vi "Dashboard Loop.vi"(10 "connection ID":refnum<k16>) -> ()   [LabVIEW 2016]
uses:
  Common Code/Intake Mode.ctl
  Common Code/Intake Commands.ctl
  Common Code/Intake Status Cluster.ctl
  Common Code/Climb Status Cluster.ctl
  Common Code/Drive Mode.ctl
  Common Code/Drivetrain Status Cluster.ctl
  Common Code/Dash Display Data.ctl
  Robot Global Data.vi
panel:
  out "length":i32
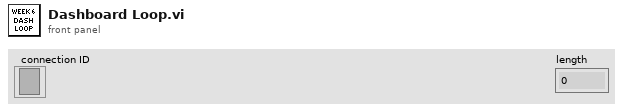
[diagram p1: front panel]
types:
  T1 = typedef "Dash Display Data.ctl" = cluster{"Intake Status Cluster ":T2, "Climb Status Cluster":T5, "Drivetrain Status Cluster":T6}
  T2 = typedef "Intake Status Cluster.ctl" = cluster{"Intake Power":dbl, "Intake Mode":T3, "Intake Command":T4}
  T3 = typedef "Intake Mode.ctl" = enum16{"Manual", "Auto"}
  T4 = typedef "Intake Commands.ctl" = enum16{"Idle", "Intake", "Outtake"}
  T5 = typedef "Climb Status Cluster.ctl" = cluster{"Power":dbl}
  T6 = typedef "Drivetrain Status Cluster.ctl" = cluster{"Gyro In Range?":bool, "Turn Power":dbl, "Steer ":dbl, "Y Power":dbl, "Drive Mode ":T7}
  T7 = typedef "Drive Mode.ctl" = enum16{"Gyro Steer", "Manual"}
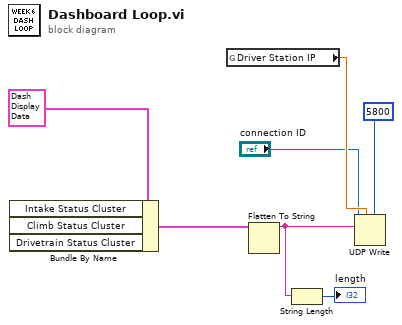
[diagram p0: block diagram]
diagram:
  n1 = Bundle By Name(cluster=T1 {"Intake Status Cluster "={"Intake Power"=0.0, "Intake Mode"=enum."Manual", "Intake Command"=enum."Idle"}, "Climb Status Cluster"={"Power"=0.0}, "Drivetrain Status Cluster"={"Gyro In Range?"=FALSE, "Turn Power"=0.0, "Steer "=0.0, "Y Power"=0.0, "Drive Mode "=enum."Gyro Steer"}} ("Dashboard Display Data")) -> (w6:T1)  [unwired: 3 in]
  n2 = global read "Robot Global Data.vi" "Driver Station IP"() -> (w4:dbl)
  n3 = Flatten To String(anything=w6) -> (data string=w2:string)  [unwired: 3 in, 2 out]
  n4 = String Length(string=w2) -> (length=→"length":i32)
  n5 = UDP Write(address=w4, port or service name=u16 5800, connection ID="connection ID", data in=w2) -> ()  [unwired: 2 in, 2 out]
